vi "ADIS16448 IMU Calibration.vi"(3 "error in":errorcluster, 5 "ADI IMU Interrupt DevRef In":T1={"ADI IMU DevRef"={"DevStatus"={"status"=FALSE, "code"=0, "source"=""}, "Handle"=0, "SPI Bus"=enum."SPI On-Board, CS0", "Device Found"=FALSE, "Device Ready"=FALSE, "Yaw Axis"=enum."Z", "AHRS Algorithm"=enum."Complementary", "Serial"=0, "Lot ID 2"=0, "Lot ID 1"=0, "Product ID"=0}, "InterruptRef"={"DevStatus"={"status"=FALSE, "code"=0, "source"=""}, "InterruptIndex"=enum."0"}}) -> (0 "error out":errorcluster, 2 "ADI IMU Interrupt DevRef Out":T1={"ADI IMU DevRef"={"DevStatus"={"status"=FALSE, "code"=0, "source"=""}, "Handle"=0, "SPI Bus"=enum."SPI On-Board, CS0", "Device Found"=FALSE, "Device Ready"=FALSE, "Yaw Axis"=enum."Z", "AHRS Algorithm"=enum."Complementary", "Serial"=0, "Lot ID 2"=0, "Lot ID 1"=0, "Product ID"=0}, "InterruptRef"={"DevStatus"={"status"=FALSE, "code"=0, "source"=""}, "InterruptIndex"=enum."0"}})   [LabVIEW 2016]
uses:
  ADI MXP IMU/WPI_IMU_ADIS16448_InterruptDevRef.ctl
  ADI MXP IMU/WPI_IMU_ADIS16448_IMUDevRef.ctl
  <vilib>/Rock Robotics/SystemInterfaces/spilib/spi_bus.ctl
  <vilib>/Rock Robotics/WPI/Interrupt/WPI_InterruptRef.ctl
  <vilib>/Rock Robotics/SystemInterfaces/Interrupt/FPGA_InterruptIndex.ctl
  <vilib>/Rock Robotics/WPI/SPI/WPI_SPIDevRef.ctl
  ADI MXP IMU/WPI_IMU_ADIS16448_Registers.ctl
  ADI MXP IMU/FRC_ADIS16448_IMU.lvlib
panel:
  out "Offset Registers":T6 {"zGYRO_OFF" format="%x"; "yGYRO_OFF" format="%x"; "xGYRO_OFF" format="%x"}
  out "Write Successful?":bool
  out "Timer":i32
  out "Device Found":bool
  # "FRC Analog Devices ADIS16448 IMU\nOffset Calibration Program"
  # "Instructions: \n* Place your robot in a stable location where it will not be bumped or moved.\n* Make sure that the IMU is securely mounted to the RoboRIO! \n* When ready, start the VI. The program will enable averaging inside of the IMU and will calculate the bias offset. \n* After recording data, the VI will save the data within the sensor for future use. \n* Running this utility again will overwrite the bias correction ."
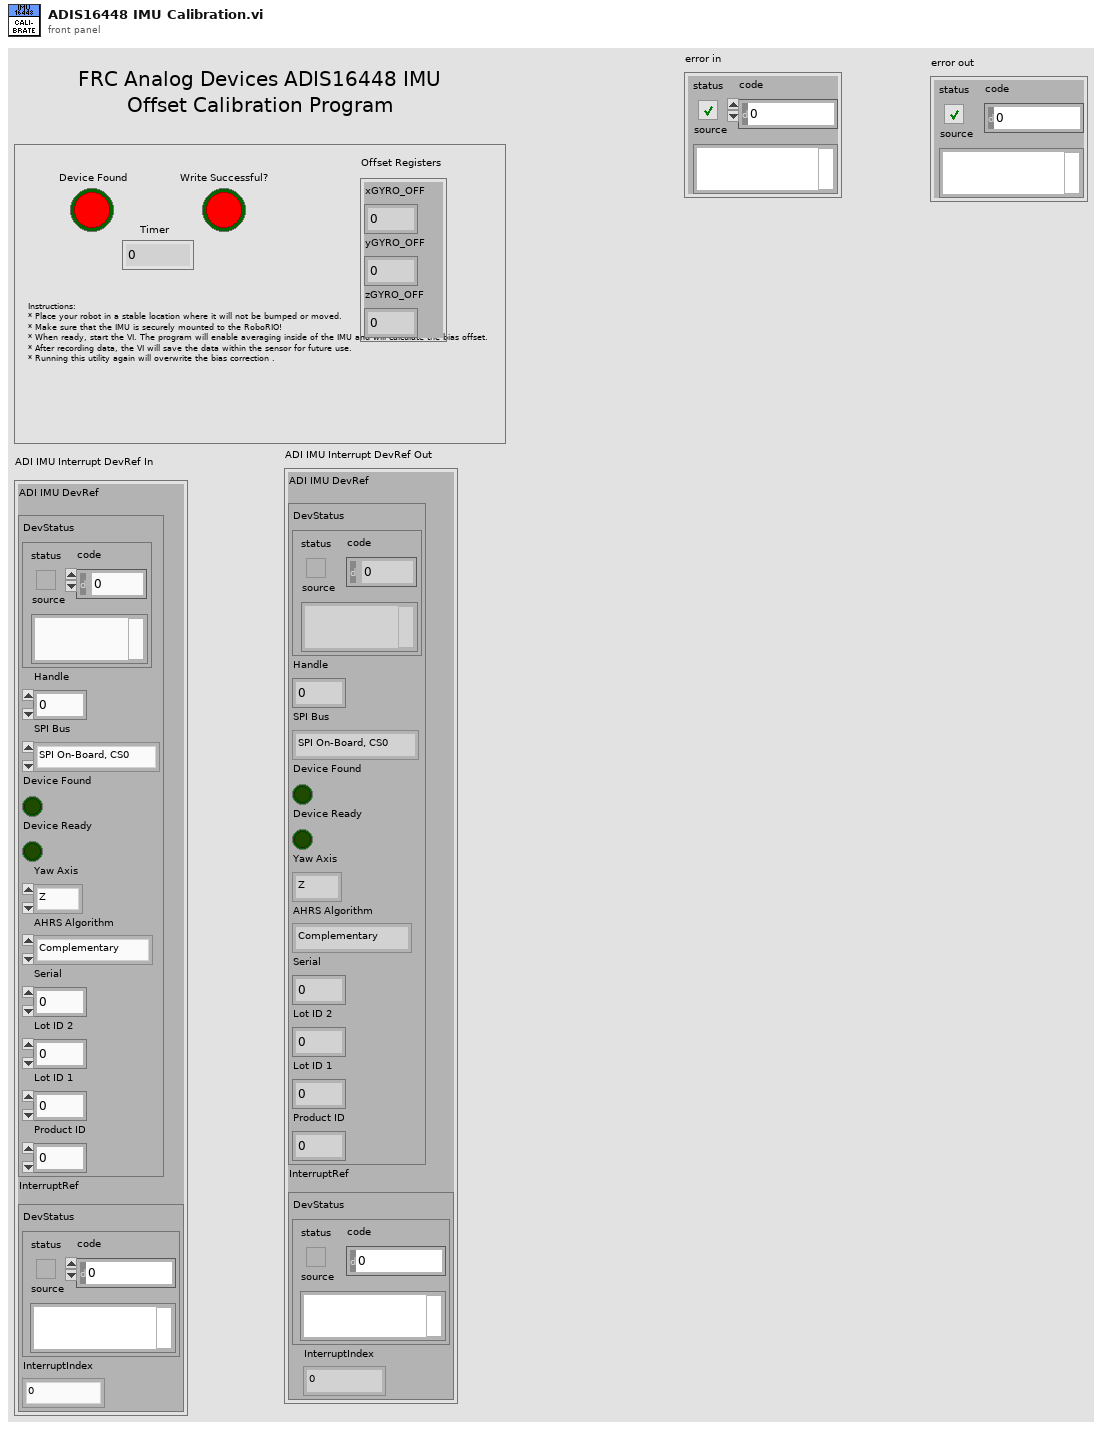
[diagram p1: front panel]
types:
  T1 = typedef "FRC_ADIS16448_IMU.lvlib/WPI_IMU_ADIS16448_InterruptDevRef.ctl" = cluster{"ADI IMU DevRef":T2, "InterruptRef":T4}
  T2 = typedef "FRC_ADIS16448_IMU.lvlib/WPI_IMU_ADIS16448_IMUDevRef.ctl" = cluster{"DevStatus":errorcluster, "Handle":i32, "SPI Bus":T3, "Device Found":bool, "Device Ready":bool, "Yaw Axis":enum16{"X", "Y", "Z"}, "AHRS Algorithm":enum16{"Complementary", "Madgwick"}, "Serial":u16, "Lot ID 2":u16, "Lot ID 1":u16, "Product ID":u16}
  T3 = typedef "spi_bus.ctl" = enum16{"SPI On-Board, CS0", "SPI On-Board, CS1", "SPI On-Board, CS2", "SPI On-Board, CS3", "SPI MXP", "Invalid"}
  T4 = typedef "WPI_InterruptRef.ctl" = cluster{"DevStatus":errorcluster, "InterruptIndex":T5}
  T5 = typedef "FPGA_InterruptIndex.ctl" = enum8{"0", "1", "2", "3", "4", "5", "6", "7", "Invalid"}
  T6 = cluster{"xGYRO_OFF":u16, "yGYRO_OFF":u16, "zGYRO_OFF":u16}
  T7 = typedef "WPI_SPIDevRef.ctl" = cluster{"DevStatus":errorcluster, "Handle":i32, "SPI Bus":T3}
  T8 = typedef "FRC_ADIS16448_IMU.lvlib/WPI_IMU_ADIS16448_Registers.ctl" = u8
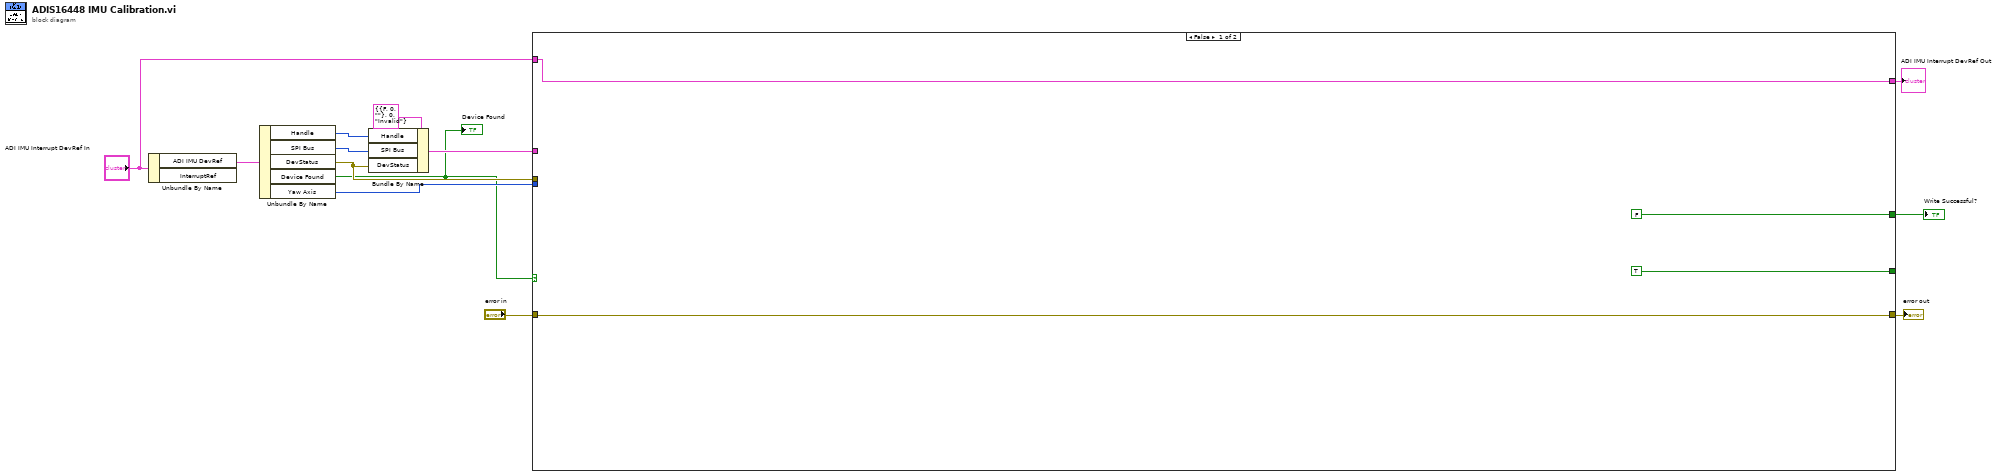
[diagram p0: block diagram]
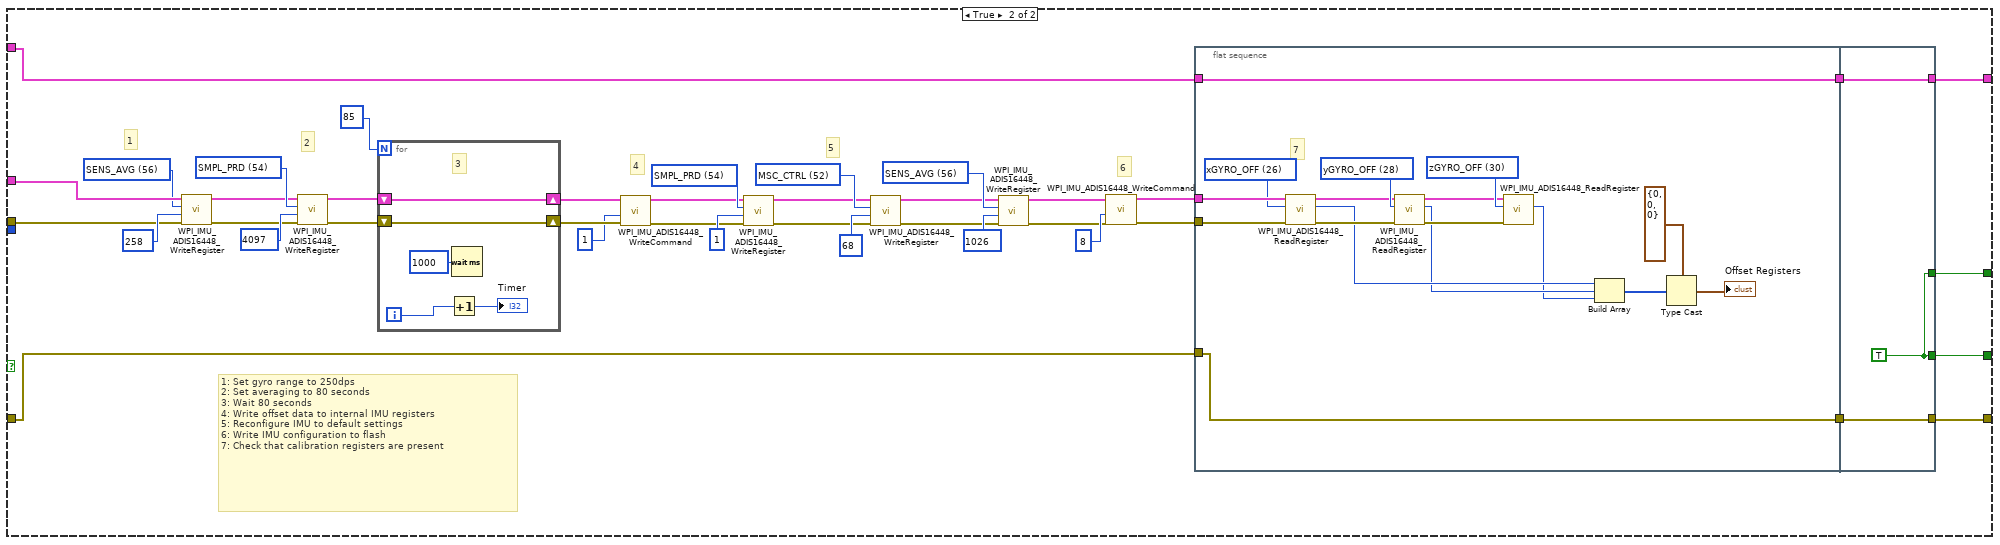
[diagram p2: hidden frame]
diagram:
  n1 = Unbundle By Name("ADI IMU Interrupt DevRef In") -> ("ADI IMU DevRef"=w10:T2)  [unwired: 1 out]
  n2 = Unbundle By Name(w10) -> ("Handle"=w12:i32, "SPI Bus"=w11:T3, "DevStatus"=w7:errorcluster, "Device Found"=w5:bool, "Yaw Axis"=w8:enum16{"X", "Y", "Z"})
  "Device Found" <- w5
  n3 = Bundle By Name(cluster=T7 {"DevStatus"={"status"=FALSE, "code"=0, "source"=""}, "Handle"=0, "SPI Bus"=enum."Invalid"} ("SPIDevRef out"), "Handle"=w12, "SPI Bus"=w11, "DevStatus"=w7) -> (w9:T7)
  n4 = case shown="False" w5 {
    tunnel: w9 -> [_ w56]
    tunnel: w8 -> [_ _]
    tunnel: w7 -> [_ w53]
    tunnel: [TRUE w37] -> _
    tunnel: [FALSE w24] -> w6
    tunnel: "ADI IMU Interrupt DevRef In" -> [w15 w23]
    tunnel: [w15 w21] -> w3
    tunnel: "error in" -> [w14 w20]
    tunnel: [w14 w18] -> w1
    frame False {
    }
    frame True {
      w40 = T8 56 items=["GLOB_CMD"=62, "SEQ_CNT"=58, "SMPL_PRD"=54, "SENS_AVG"=56, "MSC_CTRL"=52, "ERROR_FLAGS"=60, "TEMP"=44, "BARO"=40, "Z_MAG"=36, "Y_MAG"=32, "X_MAG"=28, "Z_ACCEL"=24, "Y_ACCEL"=20, "X_ACCEL"=16, "Z_GYRO"=12, "Y_GYRO"=8, "X_GYRO"=4, "PROD_ID"=86, "LOT_ID2"=84, "LOT_ID1"=82, "SERIAL_NUM"=88] ("ADIS16448 Register")
      w41 = T8 52 items=["GLOB_CMD"=62, "SEQ_CNT"=58, "SMPL_PRD"=54, "SENS_AVG"=56, "MSC_CTRL"=52, "ERROR_FLAGS"=60, "TEMP"=44, "BARO"=40, "Z_MAG"=36, "Y_MAG"=32, "X_MAG"=28, "Z_ACCEL"=24, "Y_ACCEL"=20, "X_ACCEL"=16, "Z_GYRO"=12, "Y_GYRO"=8, "X_GYRO"=4, "PROD_ID"=86, "LOT_ID2"=84, "LOT_ID1"=82, "SERIAL_NUM"=88] ("ADIS16448 Register")
      w39 = T8 54 items=["GLOB_CMD"=62, "SEQ_CNT"=58, "SMPL_PRD"=54, "SENS_AVG"=56, "MSC_CTRL"=52, "ERROR_FLAGS"=60, "TEMP"=44, "BARO"=40, "Z_MAG"=36, "Y_MAG"=32, "X_MAG"=28, "Z_ACCEL"=24, "Y_ACCEL"=20, "X_ACCEL"=16, "Z_GYRO"=12, "Y_GYRO"=8, "X_GYRO"=4, "PROD_ID"=86, "LOT_ID2"=84, "LOT_ID1"=82, "SERIAL_NUM"=88] ("ADIS16448 Register")
      w52 = T8 54 items=["GLOB_CMD"=62, "SEQ_CNT"=58, "SMPL_PRD"=54, "SENS_AVG"=56, "MSC_CTRL"=52, "ERROR_FLAGS"=60, "TEMP"=44, "BARO"=40, "Z_MAG"=36, "Y_MAG"=32, "X_MAG"=28, "Z_ACCEL"=24, "Y_ACCEL"=20, "X_ACCEL"=16, "Z_GYRO"=12, "Y_GYRO"=8, "X_GYRO"=4, "PROD_ID"=86, "LOT_ID2"=84, "LOT_ID1"=82, "SERIAL_NUM"=88] ("ADIS16448 Register")
      w55 = T8 56 items=["GLOB_CMD"=62, "SEQ_CNT"=58, "SMPL_PRD"=54, "SENS_AVG"=56, "MSC_CTRL"=52, "ERROR_FLAGS"=60, "TEMP"=44, "BARO"=40, "Z_MAG"=36, "Y_MAG"=32, "X_MAG"=28, "Z_ACCEL"=24, "Y_ACCEL"=20, "X_ACCEL"=16, "Z_GYRO"=12, "Y_GYRO"=8, "X_GYRO"=4, "PROD_ID"=86, "LOT_ID2"=84, "LOT_ID1"=82, "SERIAL_NUM"=88] ("ADIS16448 Register")
      # "5"
      # "6"
      # "4"
      # "2"
      # "1"
      # "1: Set gyro range to 250dps\n2: Set averaging to 80 seconds\n3: Wait 80 seconds\n4: Write offset data to internal IMU registers\n5: Reconfigure IMU to default settings\n6: Write IMU configuration to flash\n7: Check that calibration registers are present"
      n5 = call "WPI_IMU_ADIS16448_WriteRegister.vi"("error in (no error)"=w53, "Data"=u16 258, "ADIS16448 Register"=w55, "SPIDevRef in"=w56) -> ("error out"=w35:errorcluster, "SPIDevRef out"=w36:T7)  [unwired: 6 in]
      n6 = call "WPI_IMU_ADIS16448_WriteRegister.vi"("error in (no error)"=w35, "Data"=u16 4097, "ADIS16448 Register"=w52, "SPIDevRef in"=w36) -> ("error out"=w48:errorcluster, "SPIDevRef out"=w49:T7)  [unwired: 6 in]
      n7 = for {
        N: 85 -> [_]
        shift-right: [w80] -> w47
        shift-left: w49 -> [w80]
        shift-right: [w79] -> w46
        shift-left: w48 -> [w79]
        i -> [w77]
        # "3"
        n8 = Increment(x=w77) -> (x+1=→"Timer":i32)
        n9 = Wait (ms)(milliseconds to wait=u32 1000) -> ()  [unwired: 1 out]
      }
      n10 = call "WPI_IMU_ADIS16448_WriteCommand.vi"("error in (no error)"=w46, "Data"=u16 1, "SPIDevRef in"=w47) -> ("error out"=w33:errorcluster, "SPIDevRef out"=w34:T7)  [unwired: 7 in]
      n11 = call "WPI_IMU_ADIS16448_WriteRegister.vi"("error in (no error)"=w33, "Data"=u16 1, "ADIS16448 Register"=w39, "SPIDevRef in"=w34) -> ("error out"=w29:errorcluster, "SPIDevRef out"=w30:T7)  [unwired: 6 in]
      n12 = call "WPI_IMU_ADIS16448_WriteRegister.vi"("error in (no error)"=w29, "Data"=u16 68, "ADIS16448 Register"=w41, "SPIDevRef in"=w30) -> ("error out"=w31:errorcluster, "SPIDevRef out"=w32:T7)  [unwired: 6 in]
      n13 = call "WPI_IMU_ADIS16448_WriteRegister.vi"("error in (no error)"=w31, "Data"=u16 1026, "ADIS16448 Register"=w40, "SPIDevRef in"=w32) -> ("error out"=w27:errorcluster, "SPIDevRef out"=w28:T7)  [unwired: 6 in]
      n14 = call "WPI_IMU_ADIS16448_WriteCommand.vi"("error in (no error)"=w27, "Data"=u16 8, "SPIDevRef in"=w28) -> ("error out"=w25:errorcluster, "SPIDevRef out"=w26:T7)  [unwired: 7 in]
      n15 = flat-sequence {
        tunnel: w26 -> [w73]
        tunnel: w25 -> [w72]
        tunnel: w23 -> [w58]
        tunnel: [w58] -> w22
        tunnel: w20 -> [w57]
        tunnel: [w57] -> w19
        tunnel: [w76] -> w37
        tunnel: [w76] -> w24
        tunnel: w22 -> [w75]
        tunnel: [w75] -> w21
        tunnel: w19 -> [w74]
        tunnel: [w74] -> w18
        frame #0 {
          w69 = T8 30 items=["zGYRO_OFF"=30, "yGYRO_OFF"=28, "xGYRO_OFF"=26, "GLOB_CMD"=62, "SEQ_CNT"=58, "SMPL_PRD"=54, "SENS_AVG"=56, "MSC_CTRL"=52, "zACCEL_OFF"=36, "yACCEL_OFF"=34, "xACCEL_OFF"=32, "ERROR_FLAGS"=60, "TEMP"=24, "BARO"=22, "Z_MAG"=20, "Y_MAG"=18, "X_MAG"=16, "Z_ACCEL"=14, "Y_ACCEL"=12, "X_ACCEL"=10, "Z_GYRO"=8, "Y_GYRO"=6, "X_GYRO"=4, "PROD_ID"=86, "LOT_ID2"=84, "LOT_ID1"=82, "SERIAL_NUM"=88] ("ADIS16448 Register")
          w70 = T8 28 items=["zGYRO_OFF"=30, "yGYRO_OFF"=28, "xGYRO_OFF"=26, "GLOB_CMD"=62, "SEQ_CNT"=58, "SMPL_PRD"=54, "SENS_AVG"=56, "MSC_CTRL"=52, "zACCEL_OFF"=36, "yACCEL_OFF"=34, "xACCEL_OFF"=32, "ERROR_FLAGS"=60, "TEMP"=24, "BARO"=22, "Z_MAG"=20, "Y_MAG"=18, "X_MAG"=16, "Z_ACCEL"=14, "Y_ACCEL"=12, "X_ACCEL"=10, "Z_GYRO"=8, "Y_GYRO"=6, "X_GYRO"=4, "PROD_ID"=86, "LOT_ID2"=84, "LOT_ID1"=82, "SERIAL_NUM"=88] ("ADIS16448 Register")
          w71 = T8 26 items=["zGYRO_OFF"=30, "yGYRO_OFF"=28, "xGYRO_OFF"=26, "GLOB_CMD"=62, "SEQ_CNT"=58, "SMPL_PRD"=54, "SENS_AVG"=56, "MSC_CTRL"=52, "zACCEL_OFF"=36, "yACCEL_OFF"=34, "xACCEL_OFF"=32, "ERROR_FLAGS"=60, "TEMP"=24, "BARO"=22, "Z_MAG"=20, "Y_MAG"=18, "X_MAG"=16, "Z_ACCEL"=14, "Y_ACCEL"=12, "X_ACCEL"=10, "Z_GYRO"=8, "Y_GYRO"=6, "X_GYRO"=4, "PROD_ID"=86, "LOT_ID2"=84, "LOT_ID1"=82, "SERIAL_NUM"=88] ("ADIS16448 Register")
          # "7"
          n16 = call "WPI_IMU_ADIS16448_ReadRegister.vi"("error in (no error)"=w72, "ADIS16448 Register"=w71, "SPIDevRef in"=w73) -> ("error out"=w67:errorcluster, "Register Value"=w64:u16, "SPIDevRef out"=w68:T7)  [unwired: 6 in]
          n17 = call "WPI_IMU_ADIS16448_ReadRegister.vi"("error in (no error)"=w67, "ADIS16448 Register"=w70, "SPIDevRef in"=w68) -> ("error out"=w65:errorcluster, "Register Value"=w63:u16, "SPIDevRef out"=w66:T7)  [unwired: 6 in]
          n18 = call "WPI_IMU_ADIS16448_ReadRegister.vi"("error in (no error)"=w65, "ADIS16448 Register"=w69, "SPIDevRef in"=w66) -> ("Register Value"=w62:u16)  [unwired: 6 in, 2 out]
          n19 = Build Array(w64, w63, w62) -> (w61:u16[])
          n20 = Type Cast(type=T6 {"xGYRO_OFF"=0, "yGYRO_OFF"=0, "zGYRO_OFF"=0} ("Offset Registers 2"), x=w61) -> (*(type *) &x=→"Offset Registers":T6)
        }
        frame #1 {
          w76 = TRUE
        }
      }
    }
  }
  "Write Successful?" <- w6
  "ADI IMU Interrupt DevRef Out" <- w3
  "error out" <- w1
